vi "Do Request.vi"(7 "Processing In":refnum<class "Processing.lvclass">, 11 "ConnectRouteController in":refnum<class "ConnectRouteController.lvclass">) -> (0 "error out":errorcluster, 5 "Processing":refnum<class "Processing.lvclass">)   [LabVIEW 2022 SP3, in "VideoMux.lvlib" / "ConnectRouteController.lvclass"]
uses:
  ConnectRouteController.lvclass
  <vilib>/IlluminatedG/IG HTTP Server/HTTP Server/Processing/Processing.lvclass
  MuxAPI/MuxAPI.lvclass
  C:/Program Files (x86)/National Instruments/LabVIEW 2022/vi.lib/IlluminatedG/IG HTTP Server/HTTP Server/Service/Service.lvclass
  <vilib>/IlluminatedG/IG HTTP Server/HTTP Server/Processing/Processing.lvclass/Processing.ctl
  ConnectRouteController.lvclass/ConnectRouteController.ctl
  <vilib>/IlluminatedG/IG HTTP Utils/HTTP Utils/Request/Request.lvclass
  <vilib>/IlluminatedG/lv-stream/URI/URI.lvclass
  <vilib>/IlluminatedG/IG HTTP Utils/HTTP Utils/Response/Response.lvclass
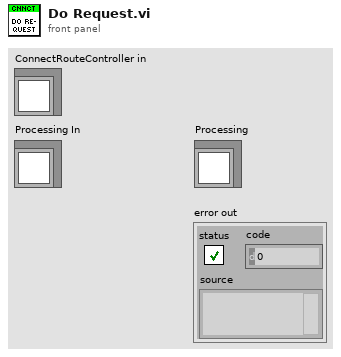
[diagram p1: front panel]
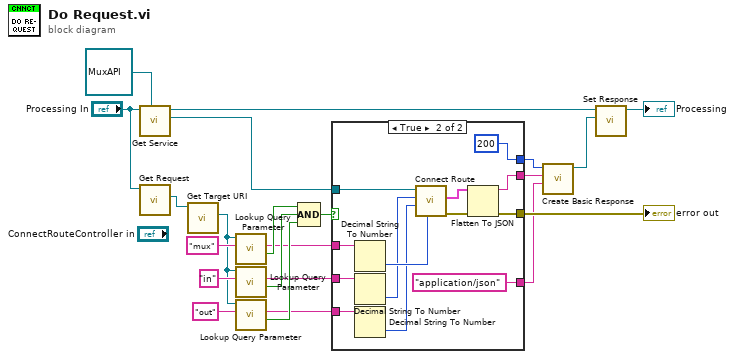
[diagram p0: block diagram]
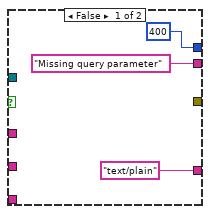
[diagram p2: hidden frame]
diagram:
  n1 = call <vilib>:"Get Service.vi"("Service Type"=refnum<class "MuxAPI.lvclass"> refnum ("VideoMux.lvlib:MuxAPI.lvclass"), "Processing in"="Processing In") -> ("Service"=w8:refnum<class "MuxAPI.lvclass">, "Processing out"=w5:refnum<class "Processing.lvclass">)  [unwired: 7 in, 1 out]
  n2 = call <vilib>:"Get Request.vi"("Processing in"="Processing In") -> ("Request"=w20:refnum<class "Request.lvclass">)  [unwired: 9 in, 1 out]
  n3 = call <vilib>:"Get Target URI.vi"("Request in"=w20) -> ("Target URI"=w16:refnum<class "URI.lvclass">)  [unwired: 8 in, 2 out]
  n4 = call <vilib>:"Lookup Query Parameter.vi"("Name"="mux", "URI in"=w16) -> ("Found"=w13:bool, "Value"=w11:string)  [unwired: 6 in, 2 out]
  n5 = call <vilib>:"Lookup Query Parameter.vi"("Name"="in", "URI in"=w16) -> ("Found"=w14:bool, "Value"=w10:string)  [unwired: 6 in, 2 out]
  n6 = call <vilib>:"Lookup Query Parameter.vi"("Name"="out", "URI in"=w16) -> ("Found"=w15:bool, "Value"=w9:string)  [unwired: 6 in, 2 out]
  n7 = Compound Arithmetic op=AND(w13, w14, w15) -> (w12:bool)
  n8 = case shown="True" w12 {
    tunnel: w11 -> [_ w38]
    tunnel: w10 -> [_ w36]
    tunnel: w9 -> [_ w37]
    tunnel: w8 -> [_ w35]
    tunnel: [_ w26] -> w7
    tunnel: [u16 400 ("Status Code") u16 200 ("Status Code")] -> w6
    tunnel: ["Missing query parameter" w29] -> w2
    tunnel: ["text/plain" ("Payload") "application/json" ("Payload")] -> w1
    frame False {
    }
    frame True {
      n9 = Decimal String To Number(string=w38) -> (number=w34:i32)  [unwired: 2 in, 1 out]
      n10 = Decimal String To Number(string=w36) -> (number=w33:i32)  [unwired: 2 in, 1 out]
      n11 = Decimal String To Number(string=w37) -> (number=w32:i32)  [unwired: 2 in, 1 out]
      n12 = call "Connect Route.vi"("Mux Index"=w34, "Output"=w32, "Input"=w33, "MuxAPI in"=w35) -> ("error out"=w27:errorcluster, "Routes"=w30:cluster{"Mux Route":i32[]}[])  [unwired: 5 in, 1 out]
      n13 = Flatten To JSON(anything=w30, error in (no error)=w27) -> (JSON string=w29:string, 11:w26:errorcluster)  [unwired: 1 in]
    }
  }
  "error out" <- w7
  n14 = call <vilib>:"Create Basic Response.vi"("Content-Type (text/plain)"=w1, "Payload"=w2, "Status Code"=w6) -> ("Response out"=w3:refnum<class "Response.lvclass">)  [unwired: 7 in, 1 out]
  n15 = call <vilib>:"Set Response.vi"("Response"=w3, "Processing in"=w5) -> ("Processing out"=→"Processing":refnum<class "Processing.lvclass">)  [unwired: 9 in]
